vi "Acquire Container Lease.vi"(8 "error in (no error)":errorcluster, 9 "Lease duration in seconds (-1: infinite)":i32=-1, 10 "Container":string, 11 "Azure Session in":refnum<class "Session.lvclass">) -> (0 "error out":errorcluster, 2 "Lease ID":string, 3 "Azure Session out":refnum<class "Session.lvclass">)   [LabVIEW 2015, in "NI_Azure_Blob.lvlib"]
doc: "Request a new lease on a container."
uses:
  NI_Azure_Blob.lvlib
  Core/Session/Session.lvclass
  Core/Name Value Pair.ctl
  Lease Action.ctl
  Core/Session/Session.lvclass/Session.ctl
  Core/Session/Write Request Headers.vi
  Core/Session/Write Request Parameters.vi
  Core/Session/Write HTTP Verb.vi
  Core/Session/Write URL Suffix.vi
  Strings Global.vi
  Core/NI_Azure_Core.lvlib
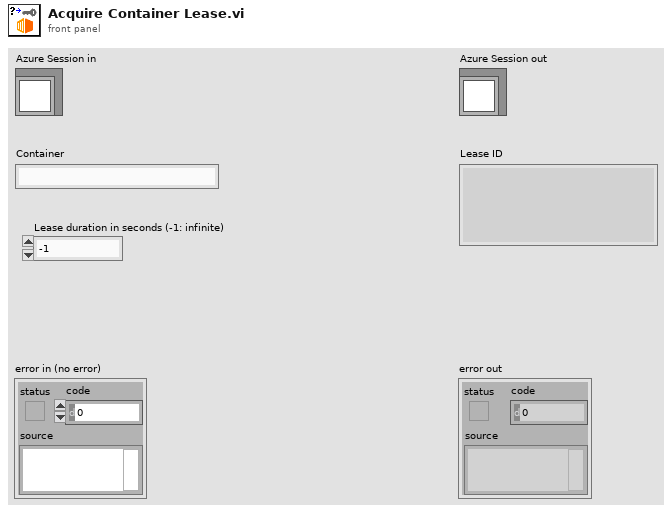
[diagram p1: front panel]
types:
  T1 = typedef "NI_Azure_Blob.lvlib/Lease Action.ctl" = enum16{"acquire", "renew", "change", "release", "break"}
  T2 = typedef "NI_Azure_Core.lvlib/Name Value Pair.ctl" = cluster{"name":string, "value":string}
  T3 = typedef "NI_Azure_Core.lvlib/Response.ctl" = cluster{"Headers":string, "Body":string}
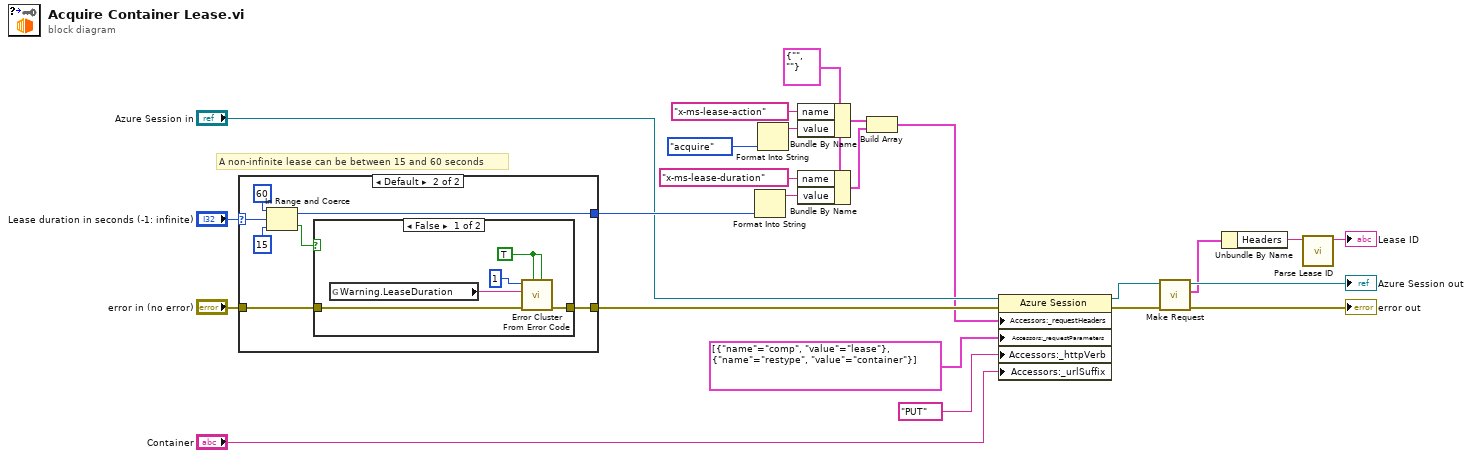
[diagram p0: block diagram]
diagram:
  w15 = T2 {"name"="", "value"=""} ("Cluster")
  # "A non-infinite lease can be between 15 and 60 seconds"
  n1 = case shown="Default" "Lease duration in seconds (-1: infinite)" {
    selector: "Lease duration in seconds (-1: infinite)" -> [w26 w31]
    tunnel: [w26 w30] -> w9
    tunnel: "error in (no error)" -> [w25 w29]
    tunnel: [w25 w28] -> w10
    frame -1 {
    }
    frame Default {
      n2 = In Range and Coerce(upper limit=60, x=w31, lower limit=15) -> (coerced(x)=w30:i32, In Range?=w27:bool)
      n3 = case shown="False" w27 {
        tunnel: w29 -> [w37 w39]
        tunnel: [w36 w39] -> w28
        frame False {
          w38 = TRUE ("show call chain? (False)")
          n4 = global read "Strings Global.vi" "Warning.LeaseDuration"() -> (w34:string)
          n5 = call <vilib>:"Error Cluster From Error Code.vi"("is warning? (False)"=w38, "show call chain? (False)"=w38, "error in (no error)"=w37, "error message (\"\")"=w34, "error code (0)"=1) -> ("error out"=w36:errorcluster)  [unwired: 4 in]
        }
        frame True {
        }
      }
    }
  }
  n6 = Format Into String(w9) -> (resulting string=w13:string)  [unwired: 3 in, 1 out]
  n7 = Format Into String(Lease_Action."acquire" ("Lease action")) -> (resulting string=w17:string)  [unwired: 3 in, 1 out]
  n8 = Bundle By Name(cluster=w15, "name"="x-ms-lease-action" ("header"), "value"=w17) -> (w19:T2)
  n9 = Bundle By Name(cluster=w15, "name"="x-ms-lease-duration" ("header"), "value"=w13) -> (w12:T2)
  n10 = Build Array(w19, w12) -> (w3:T2[])
  n11 = property class="Azure Session"(reference="Azure Session in", error in=w10, "Accessors:_requestHeaders"=w3, "Accessors:_requestParameters"=T2[] [{"name"="comp", "value"="lease"}, {"name"="restype", "value"="container"}] ("request parameters"), "Accessors:_httpVerb"="PUT" ("HTTP-Verb"), "Accessors:_urlSuffix"="Container") -> (reference out=w5:refnum<class "Session.lvclass">, error out=w7:errorcluster)
  n12 = call "Make Request.vi"("error in (no error)"=w7, "Session in"=w5) -> ("error out"=→"error out":errorcluster, "Response"=w8:T3, "Session out"=→"Azure Session out":refnum<class "Session.lvclass">)  [unwired: 7 in]
  n13 = Unbundle By Name(w8) -> ("Headers"=w11:string)
  n14 = call "Parse Lease ID.vi"("String"=w11) -> ("Lease id"=→"Lease ID":string)  [unwired: 10 in]
